vi "servoClose (SubVI).vi"(8 "Error In":errorcluster, 11 "ServosRef":refnum<class "PWM Generator.lvclass">[](array[class])) -> (0 "error out":errorcluster)   [LabVIEW 2020]
uses:
  <vilib>/CISH Robotics/L4VMX VMXpi/PWM Generator/PWM Generator.lvclass
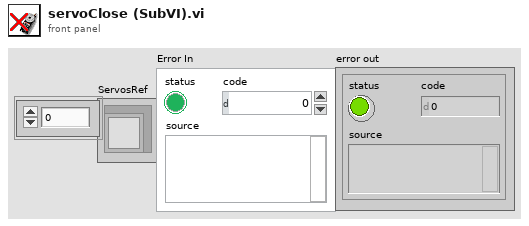
[diagram p1: front panel]
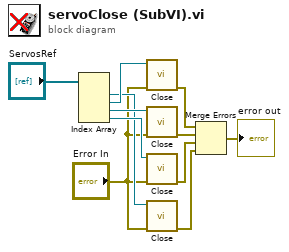
[diagram p0: block diagram]
diagram:
  n1 = Index Array(array="ServosRef") -> (element #1=w8:refnum<class "PWM Generator.lvclass">, element #2=w9:refnum<class "PWM Generator.lvclass">, element #3=w10:refnum<class "PWM Generator.lvclass">, element #4=w11:refnum<class "PWM Generator.lvclass">)  [unwired: 4 in]
  n2 = call <vilib>:"Close.vi"("Error In"="Error In", "PWM Generator Object"=w9) -> ("Error Out"=w5:errorcluster)  [unwired: 9 in]
  n3 = call <vilib>:"Close.vi"("Error In"="Error In", "PWM Generator Object"=w10) -> ("Error Out"=w4:errorcluster)  [unwired: 9 in]
  n4 = call <vilib>:"Close.vi"("Error In"="Error In", "PWM Generator Object"=w11) -> ("Error Out"=w3:errorcluster)  [unwired: 9 in]
  n5 = call <vilib>:"Close.vi"("Error In"="Error In", "PWM Generator Object"=w8) -> ("Error Out"=w2:errorcluster)  [unwired: 9 in]
  n6 = Merge Errors(w5, w4, w3, w2) -> (→"error out":errorcluster)
